vi "RunAllTests.vi"() -> ()   [LabVIEW 2019]
uses:
  ca6f43b0-97b5-4861-9fe9-a37eff1204c5.vi
  Tests.SolutionBuilder/Tests.SolutionBuilder.lvlib
  SolutionBuilder/SolutionBuilder.lvlib
panel:
  in  "Stop on Fail?":bool
  in  "Open failed tests?":bool=TRUE
  out "All Pass?":bool
  in  "Test results":i32(listbox)=-1
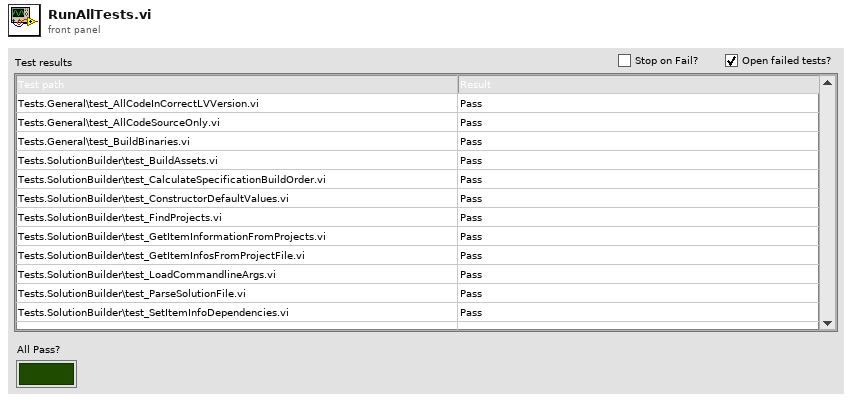
[diagram p1: front panel]
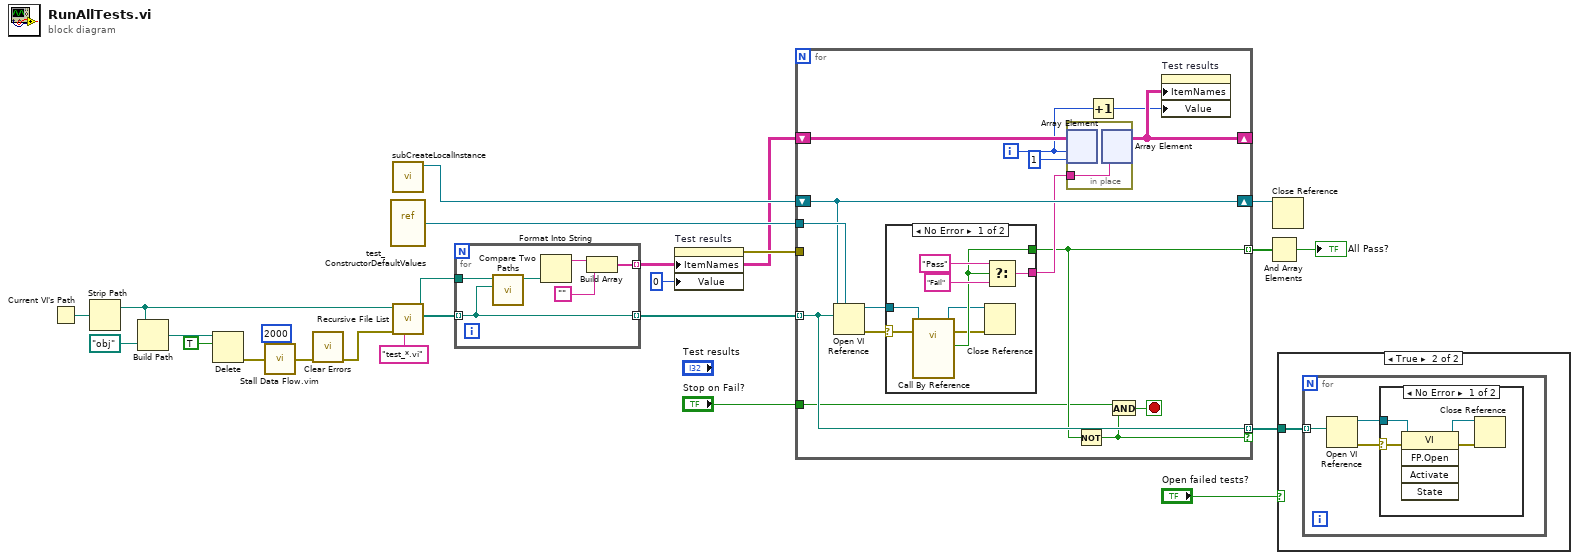
[diagram p0: block diagram]
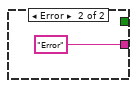
[diagram p4: hidden frame]
diagram:
  n1 = Current VI's Path() -> (path=w24:path)
  n2 = Strip Path(path=w24) -> (stripped path=w19:path)  [unwired: 1 out]
  n3 = Build Path(base path=w19, name or relative path=path "obj") -> (appended path=w17:path)
  n4 = Delete(path (use dialog)=w17, entire hierarchy (F)=TRUE) -> (error out=w15:errorcluster)  [unwired: 3 in, 2 out]
  n5 = call "Stall Data Flow.vim"("value in"=w15, "milliseconds to wait"=u32 2000) -> ("value out"=w13:errorcluster)  [unwired: 1 out]
  n6 = call <vilib>:"Clear Errors.vi"("error in (no error)"=w13) -> ("error out"=w12:errorcluster)  [unwired: 5 in, 1 out]
  n7 = vi-ref "test_ConstructorDefaultValues.vi"() -> (w22:refnum<vi>)
  n8 = call "subCreateLocalInstance.vi"() -> ("Application out"=w10:refnum<vi>)  [unwired: 11 in]
  n9 = call <vilib>:"Recursive File List.vi"("pattern"="test_*.vi", "error in (no error)"=w12, "Folder Path"=w19) -> ("All Files in Dir"=w9:path[], "dup Folder Path"=w7:path)  [unwired: 4 in, 3 out]
  n10 = for {
    tunnel: w9 -> [w28] mode=indexing
    tunnel: [w28] -> w8 mode=indexing
    tunnel: w7 -> [w29]
    tunnel: [w25] -> w4 mode=indexing
    n11 = call <vilib>:"Compare Two Paths.vi"("Path 2"=w28, "Path 1"=w29) -> ("Relative Path from 1 to 2"=w30:path)  [unwired: 6 in, 3 out]
    n12 = Format Into String(w30) -> (resulting string=w27:string)  [unwired: 3 in, 1 out]
    n13 = Build Array(w27, "") -> (w25:string[])
  }
  n14 = property on="Test results" class="MCListbox (strict)"("ItemNames"=w4, "Value"=0 ("Test results")) -> (error out=w5:errorcluster)  [unwired: 2 in, 1 out]
  n15 = for {
    tunnel: w8 -> [w37] mode=indexing
    tunnel: w22 -> [w45]
    tunnel: [w36] -> w21 mode=indexing
    shift-right: [w42] -> w11
    shift-left: w10 -> [w42]
    tunnel: w5 -> [_]
    shift-right: [w38] -> _
    shift-left: w4 -> [w41]
    tunnel: [w37] -> w2 mode=indexing if=w32
    tunnel: "Stop on Fail?" -> [w33]
    i -> [w35]
    stop <- w31 stop-if-true
    n16 = Open VI Reference(type specifier VI Refnum (for type only)=w45, application reference (local)=w42, vi path=w37) -> (vi reference=w44:refnum<vi>, error out=w43:errorcluster)  [unwired: 3 in]
    n17 = case shown="No Error" w43 {
      selector: w43 -> [w51 _]
      tunnel: w44 -> [w54 _]
      tunnel: [w49 "Error" ("resulting string")] -> w39
      tunnel: [w50 _] -> w36
      frame No Error {
        n18 = call-by-ref "?"(reference=w54, error in=w51) -> (reference out=w47:refnum<vi>, error out=w48:errorcluster, "Pass?"=w50:bool)  [unwired: 11 in]
        n19 = Close Reference(reference=w47, error in (no error)=w48) -> ()  [unwired: 1 out]
        n20 = Select(t="Pass" ("resulting string"), s=w50, f="Fail" ("resulting string")) -> (s? t:f=w49:string)
      }
      frame Error {
      }
    }
    n21 = in-place {
      in-place-border: w39 -> [w46]
      n22 = in-place-array #1(w41, w35, 1) -> ()  [unwired: 1 out]
      n23 = in-place-array #1(w46) -> (w38:string[][])  [unwired: 2 out]
    }
    n24 = Not(x=w36) -> (.not. x?=w32:bool)
    n25 = Increment(x=w35) -> (x+1=w34:i32)
    n26 = And(x=w33, y=w32) -> (x .and. y?=w31:bool)
    n27 = property on="Test results" class="MCListbox (strict)"("ItemNames"=w38, "Value"=w34) -> ()  [unwired: 2 in, 2 out]
  }
  n28 = And Array Elements(Boolean array=w21) -> (logical AND=→"All Pass?":bool)
  n29 = Close Reference(reference=w11) -> ()  [unwired: 1 in, 1 out]
  n30 = case shown="True" "Open failed tests?" {
    tunnel: w2 -> [_ w56]
    frame False {
    }
    frame True {
      n31 = for {
        tunnel: w56 -> [w57] mode=indexing
        n32 = Open VI Reference(vi path=w57) -> (vi reference=w59:refnum<vi>, error out=w58:errorcluster)  [unwired: 5 in]
        n33 = case shown="No Error" w58 {
          selector: w58 -> [w62 _]
          tunnel: w59 -> [w63 _]
          frame No Error {
            n34 = invoke class="VI" method="FP.Open"(reference=w63, error in=w62) -> (reference out=w60:refnum<vi>, error out=w61:errorcluster)  [unwired: 3 in, 3 out]
            n35 = Close Reference(reference=w60, error in (no error)=w61) -> ()  [unwired: 1 out]
          }
          frame Error {
          }
        }
      }
    }
  }
